vi "Make Segment.vi"(0 "TreeNode in":refnum<class "TreeNode.lvclass">, 1 "Start":refnum<class "Data.lvclass">, 2 "End":refnum<class "Data.lvclass">, 3 "Dimension":refnum<class "Data.lvclass">, 4 "Data":refnum<class "Array.lvclass">, 5 "error in (no error)":errorcluster) -> (14 "TreeNode out":refnum<class "TreeNode.lvclass">, 19 "error out":errorcluster)   [LabVIEW 2013, in "MDSplus.lvlib" / "TreeNode.lvclass"]
doc: "Initializes and fills a new segment."
uses:
  <vilib>/MDSplus/Classes/Data_Class/TreeNode_Class/TreeNode.lvclass
  <vilib>/MDSplus/Classes/Data_Class/Data.lvclass
  <vilib>/MDSplus/Classes/Data_Class/Array_Class/Array.lvclass
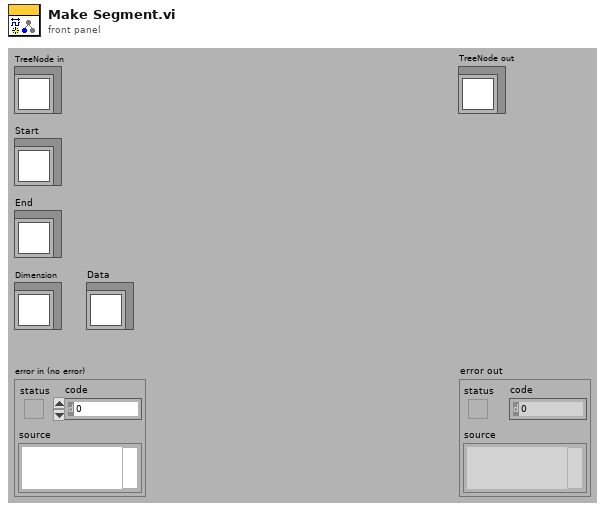
[diagram p1: front panel]
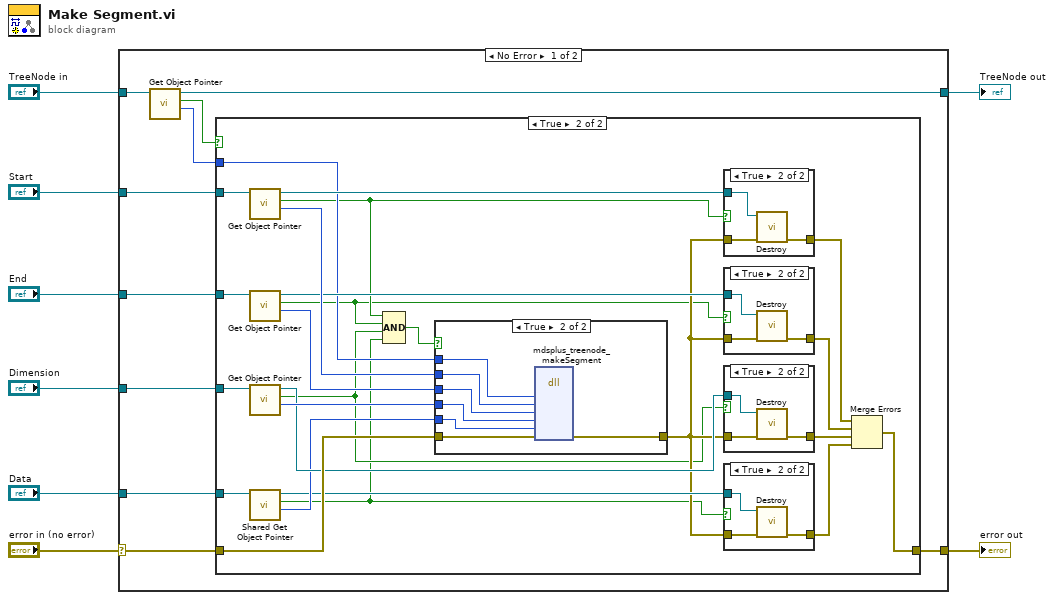
[diagram p0: block diagram]
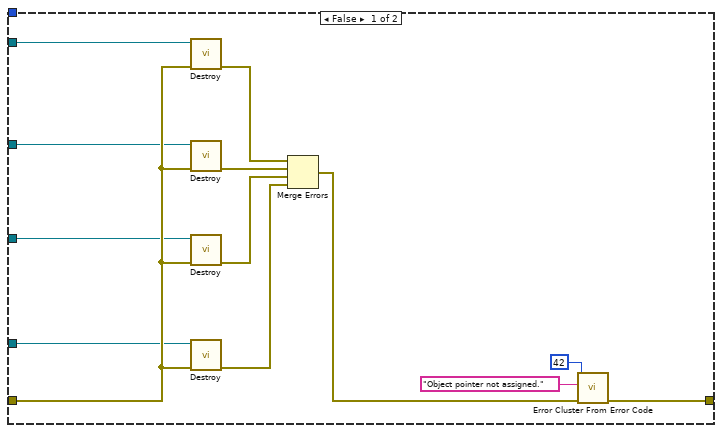
[diagram p2: hidden frame]
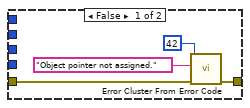
[diagram p7: hidden frame]
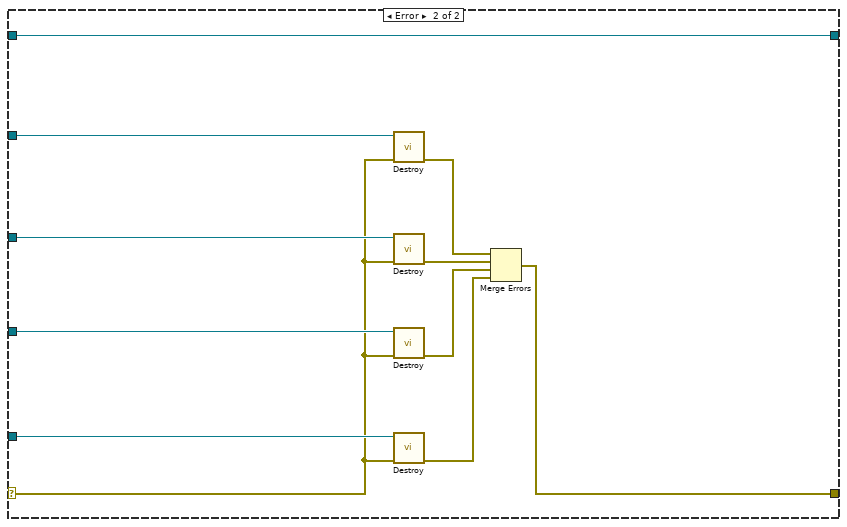
[diagram p8: hidden frame]
diagram:
  n1 = case shown="No Error" "error in (no error)" {
    selector: "error in (no error)" -> [w15 w85]
    tunnel: [w14 w87] -> w7
    tunnel: [w11 w94] -> w6
    tunnel: "TreeNode in" -> [w12 w94]
    tunnel: "Start" -> [w18 w93]
    tunnel: "End" -> [w17 w92]
    tunnel: "Dimension" -> [w16 w91]
    tunnel: "Data" -> [w13 w86]
    frame No Error {
      n2 = call-dynamic "Get Object Pointer.vi"("Data in"=w12) -> ("Object Pointer"=w9:i64, "Assigned object pointer?"=w10:bool, "Data out"=w11:refnum<class "TreeNode.lvclass">)  [unwired: 8 in]
      n3 = case shown="True" w10 {
        tunnel: w18 -> [w27 w56]
        tunnel: w17 -> [w25 w55]
        tunnel: w16 -> [w24 w54]
        tunnel: w15 -> [w26 w50]
        tunnel: [w19 w43] -> w14
        tunnel: w13 -> [w23 w42]
        tunnel: w9 -> [_ w36]
        frame False {
          n4 = call-dynamic "Destroy.vi"("error in (no error)"=w26, "Data in"=w27) -> ("error out"=w29:errorcluster)  [unwired: 9 in]
          n5 = call-dynamic "Destroy.vi"("error in (no error)"=w26, "Data in"=w25) -> ("error out"=w31:errorcluster)  [unwired: 9 in]
          n6 = call-dynamic "Destroy.vi"("error in (no error)"=w26, "Data in"=w24) -> ("error out"=w30:errorcluster)  [unwired: 9 in]
          n7 = call-dynamic "Destroy.vi"("error in (no error)"=w26, "Array in"=w23) -> ("error out"=w28:errorcluster)  [unwired: 9 in]
          n8 = Merge Errors(w29, w31, w30, w28) -> (w20:errorcluster)
          n9 = call <vilib>:"Error Cluster From Error Code.vi"("error in (no error)"=w20, "error message (\"\")"="Object pointer not assigned." ("error message (\"\")"), "error code (0)"=42) -> ("error out"=w19:errorcluster)  [unwired: 6 in]
        }
        frame True {
          n10 = call-dynamic "Get Object Pointer.vi"("Data in"=w56) -> ("Object Pointer"=w51:i64, "Assigned object pointer?"=w35:bool, "Data out"=w49:refnum<class "Data.lvclass">)  [unwired: 8 in]
          n11 = call-dynamic "Get Object Pointer.vi"("Data in"=w55) -> ("Object Pointer"=w52:i64, "Assigned object pointer?"=w34:bool, "Data out"=w48:refnum<class "Data.lvclass">)  [unwired: 8 in]
          n12 = call-dynamic "Get Object Pointer.vi"("Data in"=w54) -> ("Object Pointer"=w53:i64, "Assigned object pointer?"=w33:bool, "Data out"=w47:refnum<class "Data.lvclass">)  [unwired: 8 in]
          n13 = call <vilib>:"Shared Get Object Pointer.vi"("Data in"=w42) -> ("Object Pointer"=w41:i64, "Assigned object pointer?"=w32:bool, "Data out"=w40:refnum<class "Array.lvclass">)  [unwired: 8 in]
          n14 = Compound Arithmetic op=AND(w35, w34, w33, w32) -> (w39:bool)
          n15 = case shown="True" w39 {
            tunnel: w53 -> [_ w83]
            tunnel: w52 -> [_ w82]
            tunnel: w51 -> [_ w81]
            tunnel: w50 -> [w74 w80]
            tunnel: [w73 w79] -> w38
            tunnel: w41 -> [_ w78]
            tunnel: w36 -> [_ w77]
            frame False {
              n16 = call <vilib>:"Error Cluster From Error Code.vi"("error in (no error)"=w74, "error message (\"\")"="Object pointer not assigned." ("error message (\"\")"), "error code (0)"=42) -> ("error out"=w73:errorcluster)  [unwired: 6 in]
            }
            frame True {
              n17 = dll-call lib="MDSobjectsLVShr" fn="mdsplus_treenode_makeSegment"("lvTreeNodePtr"=w77, "lvStartDataPtrIn"=w81, "lvEndDataPtrIn"=w82, "lvTimeDataPtrIn"=w83, "lvArrPtrIn"=w78, "error"=w80) -> ("error"=w79:errorcluster)  [unwired: 9 in, 2 out]
            }
          }
          n18 = case shown="True" w35 {
            tunnel: w38 -> [w65 w68]
            tunnel: w49 -> [_ w67]
            tunnel: [w65 w66] -> w44
            frame False {
            }
            frame True {
              n19 = call-dynamic "Destroy.vi"("error in (no error)"=w68, "Data in"=w67) -> ("error out"=w66:errorcluster)  [unwired: 9 in]
            }
          }
          n20 = case shown="True" w34 {
            tunnel: w38 -> [w69 w72]
            tunnel: w48 -> [_ w71]
            tunnel: [w69 w70] -> w45
            frame False {
            }
            frame True {
              n21 = call-dynamic "Destroy.vi"("error in (no error)"=w72, "Data in"=w71) -> ("error out"=w70:errorcluster)  [unwired: 9 in]
            }
          }
          n22 = case shown="True" w33 {
            tunnel: w38 -> [w61 w64]
            tunnel: w47 -> [_ w63]
            tunnel: [w61 w62] -> w46
            frame False {
            }
            frame True {
              n23 = call-dynamic "Destroy.vi"("error in (no error)"=w64, "Data in"=w63) -> ("error out"=w62:errorcluster)  [unwired: 9 in]
            }
          }
          n24 = case shown="True" w32 {
            tunnel: w38 -> [w57 w60]
            tunnel: w40 -> [_ w59]
            tunnel: [w57 w58] -> w37
            frame False {
            }
            frame True {
              n25 = call-dynamic "Destroy.vi"("error in (no error)"=w60, "Array in"=w59) -> ("error out"=w58:errorcluster)  [unwired: 9 in]
            }
          }
          n26 = Merge Errors(w44, w45, w46, w37) -> (w43:errorcluster)
        }
      }
    }
    frame Error {
      n27 = call-dynamic "Destroy.vi"("error in (no error)"=w85, "Data in"=w93) -> ("error out"=w88:errorcluster)  [unwired: 9 in]
      n28 = call-dynamic "Destroy.vi"("error in (no error)"=w85, "Data in"=w92) -> ("error out"=w90:errorcluster)  [unwired: 9 in]
      n29 = call-dynamic "Destroy.vi"("error in (no error)"=w85, "Data in"=w91) -> ("error out"=w89:errorcluster)  [unwired: 9 in]
      n30 = call-dynamic "Destroy.vi"("error in (no error)"=w85, "Array in"=w86) -> ("error out"=w84:errorcluster)  [unwired: 9 in]
      n31 = Merge Errors(w88, w90, w89, w84) -> (w87:errorcluster)
    }
  }
  "error out" <- w7
  "TreeNode out" <- w6
